vi "Write Bool.vi"(8 "error in (no error)":errorcluster, 9 "Write Data":bool, 10 "Start address":string, 11 "MelsecTCP in":refnum<class "Abs Controler.lvclass">) -> (0 "error out":errorcluster, 3 "MelsecTCP out":refnum<class "Abs Controler.lvclass">)   [LabVIEW 2020, in "HslCommunication.lvlib" / "Abs Controler.lvclass"]
uses:
  Abs Controler.lvclass
  E:/Git/Libraries/develop/HslCommunication/_Dependenciecs/HslCommunication.dll
  _Dependenciecs/HslCommunication.dll
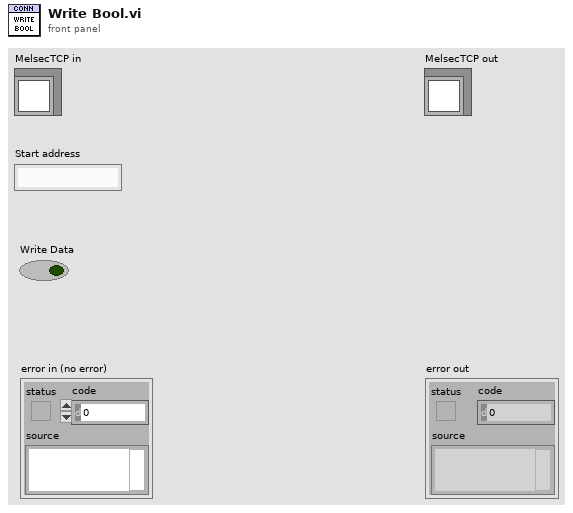
[diagram p1: front panel]
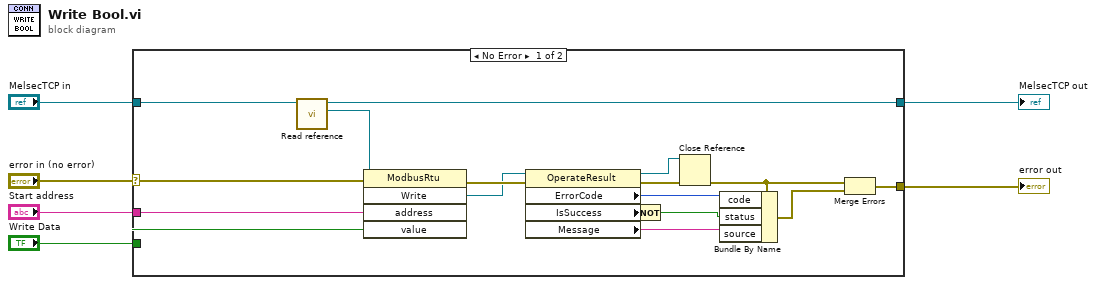
[diagram p0: block diagram]
diagram:
  n1 = case shown="No Error" "error in (no error)" {
    selector: "error in (no error)" -> [w19 w25]
    tunnel: "MelsecTCP in" -> [w22 w24]
    tunnel: [w23 w24] -> w1
    tunnel: "Start address" -> [w21 _]
    tunnel: [w20 w25] -> w3
    tunnel: "Write Data" -> [w8 _]
    frame No Error {
      n2 = call-dynamic "Read reference.vi"("Abs Controler in"=w22) -> ("reference"=w7:refnum<k24>, "Abs Controler out"=w23:refnum<class "Abs Controler.lvclass">)  [unwired: 8 in, 1 out]
      n3 = invoke class="ModbusRtu" method="Write"(reference=w7, error in=w19, "address"=w21, "value"=w8) -> (error out=w13:errorcluster, "Write"=w11:refnum<k24>)  [unwired: 1 in, 3 out]
      n4 = property class="OperateResult"(reference=w11, error in=w13) -> (reference out=w10:refnum<k24>, error out=w12:errorcluster, "ErrorCode"=w18:i32, "IsSuccess"=w17:bool, "Message"=w16:string)
      n5 = Not(x=w17) -> (.not. x?=w9:bool)
      n6 = Close Reference(reference=w10, error in (no error)=w12) -> (error out=w15:errorcluster)
      n7 = Bundle By Name(cluster=w15, "code"=w18, "status"=w9, "source"=w16) -> (w14:errorcluster)
      n8 = Merge Errors(w15, w14) -> (w20:errorcluster)
    }
    frame Error {
    }
  }
  "error out" <- w3
  "MelsecTCP out" <- w1
